vi "invalidate bad data timestamps.vi"(7 "sample counter":i32, 8 "error in":errorcluster, 10 "cache allocation in":T1, 11 "bin file in":refnum<file>) -> (0 "error out":errorcluster, 2 "cache allocation out":T1, 3 "bin file out":refnum<file>)   [LabVIEW 2013, in "Binary datalogger runtime.lvclass"]
uses:
  Binary datalogger runtime.lvclass
  data cache.ctl
  <vilib>/NI/Tag Bus/table/data table.ctl
  <vilib>/NI/Tag Bus/table/data table.lvlib
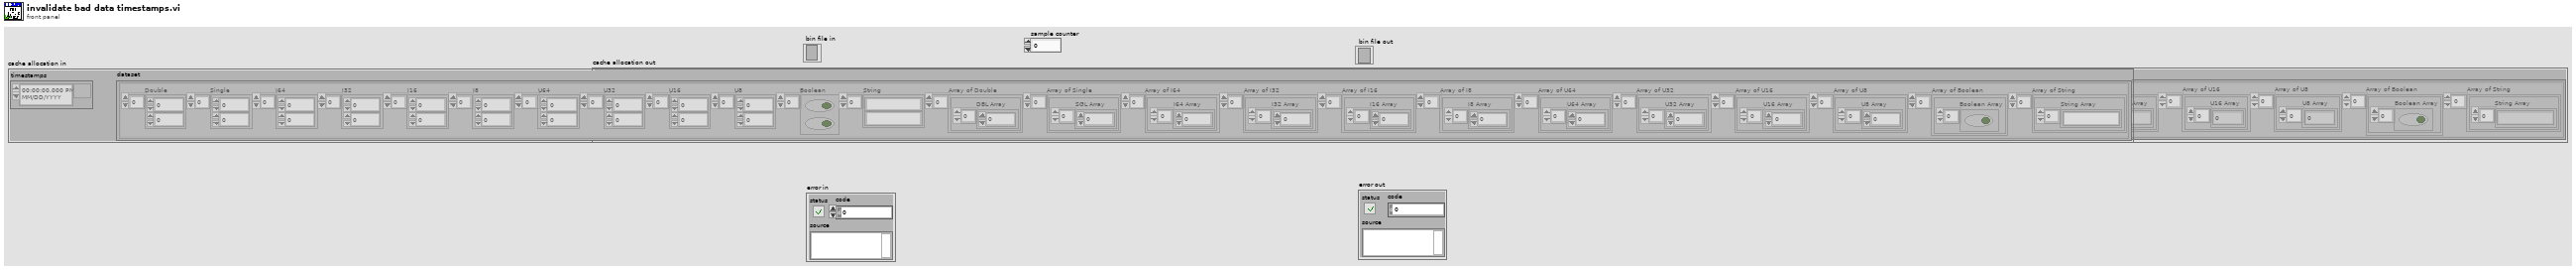
[diagram p1: front panel]
types:
  T1 = typedef "Binary datalogger runtime.lvclass/data cache.ctl" = cluster{"timestamps":timestamp[], "dataset":T2[]}
  T2 = typedef "tag bus.lvlib/data table.lvlib/data table.ctl" = cluster{"Double":dbl[], "Single":sgl[], "I64":i64[], "I32":i32[], "I16":i16[], "I8":i8[], "U64":u64[], "U32":u32[], "U16":u16[], "U8":u8[], "Boolean":bool[], "String":string[], "Array of Double":cluster{"DBL Array":dbl[]}[], "Array of Single":cluster{"SGL Array":sgl[]}[], "Array of I64":cluster{"I64 Array":i64[]}[], "Array of I32":cluster{"I32 Array":i32[]}[], "Array of I16":cluster{"I16 Array":i16[]}[], "Array of I8":cluster{"I8 Array":i8[]}[], "Array of U64":cluster{"U64 Array":u64[]}[], "Array of U32":cluster{"U32 Array":u32[]}[], "Array of U16":cluster{"U16 Array":u16[]}[], "Array of U8":cluster{"U8 Array":u8[]}[], "Array of Boolean":cluster{"Boolean Array":bool[]}[], "Array of String":cluster{"String Array":string[]}[]}
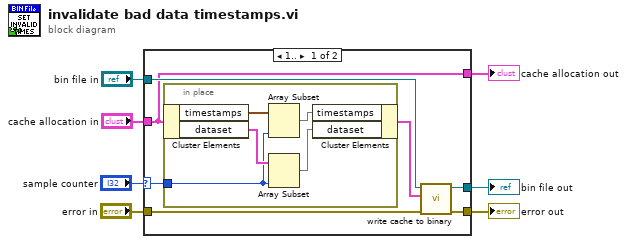
[diagram p0: block diagram]
diagram:
  n1 = case shown="1.." "sample counter" {
    selector: "sample counter" -> [w8 _]
    tunnel: "cache allocation in" -> [w9 w20]
    tunnel: "error in" -> [w14 w21]
    tunnel: "bin file in" -> [w13 w22]
    tunnel: [w12 w22] -> w3
    tunnel: [w11 w21] -> w2
    tunnel: [w9 w20] -> w1
    frame 1.. {
      n2 = in-place {
        in-place-border: w8 -> [w15]
        n3 = in-place-cluster #1(w9) -> ("timestamps"=w16:timestamp[], "dataset"=w19:T2[])
        n4 = Array Subset(array=w16, length=w15) -> (w17:timestamp[])  [unwired: 1 in]
        n5 = Array Subset(array=w19, length=w15) -> (w18:T2[])  [unwired: 1 in]
        n6 = in-place-cluster #1("timestamps"=w17, "dataset"=w18) -> (w10:T1)
      }
      n7 = call "write cache to binary.vi"("error in"=w14, "cache in"=w10, "bin file in"=w13) -> ("error out"=w11:errorcluster, "bin file out"=w12:refnum<file>)  [unwired: 6 in, 1 out]
    }
    frame 0, Default {
    }
  }
  "cache allocation out" <- w1
  "bin file out" <- w3
  "error out" <- w2
